vi "QTrkTest.vi"() -> ()   [LabVIEW 2015]
uses:
  QTrkLVBinding/QTrkSettings.ctl
  QTrkLVBinding/QTrkLocalizationType.ctl
  QTrkLVBinding/QTrkZCommandType.ctl
  QTrkLVBinding/QTrkDLL.vi
panel:
  in  "Number of ZLUTs":i32=1
  in  "Select dll":bool
  out "Sample img":sgl[][](graph)
  in  "stop test":bool
  out "Frame#":i32
  out "Frames/s":dbl
  in  "Testing sample count":i32=10000
  out "testing results":i32
  out "Single ZLUT plane image":sgl[][](graph)
  in  "Run":bool
  in  "stop":bool
  in  "LUT radii":cluster{"min":sgl, "max":sgl}={"min"=0.0, "max"=40.0}
  out "LUT":u8[][](graph)
  out "Generated LUT":sgl[][](graph)
  in  "Max Z":dbl=180.0
  in  "Min Z":dbl
  in  "QTrk Settings":T1={"Image width"=80, "Image height"=80, "Number of threads (CPU based)"=-1, "CUDA Device"=128, "COM Background correction factor"=2.0, "ZLUT MinRadius"=2.0, "ZLUT Radial sample density"=30.0, "ZLUT Angular sample density"=128.0, "ZLUT ROI Coverage"=32.0, "QI Iterations"=4, "QI MinRadius"=2.0, "QI Radial sample density"=32.0, "QI Angular sample density"=30.0, "QI ROI Coverage"=0.0, "QI Angular Step \nIteration Factor"=32.0, "XCOR Profile Length"=32, "XCOR Profile Width"=2, "XCOR Iterations"=5, "Gaussian 2D Fit Iterations"=8, "Gaussian 2D Sigma (pixels)"=3.0, "Downsample"=0}
  # "-2: Use all devices\n-1: Use best device"
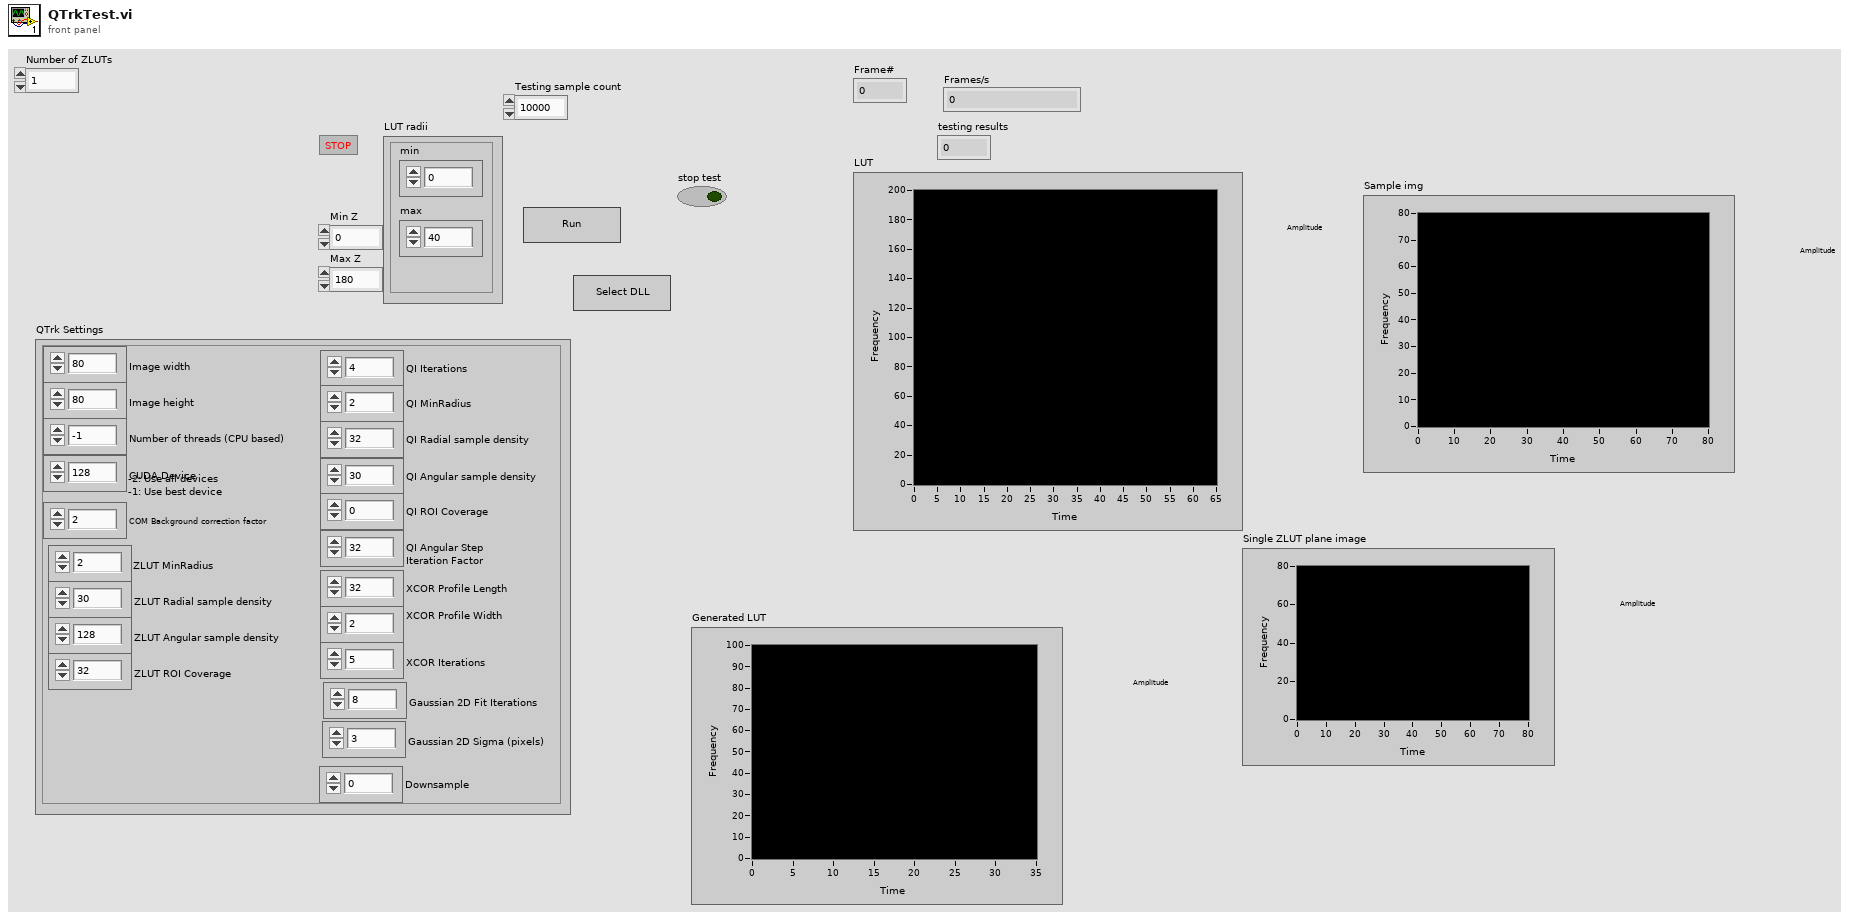
[diagram p1: front panel]
types:
  T1 = typedef "QTrkSettings.ctl" = cluster{"Image width":i32, "Image height":i32, "Number of threads (CPU based)":i32, "CUDA Device":i32, "COM Background correction factor":sgl, "ZLUT MinRadius":sgl, "ZLUT Radial sample density":sgl, "ZLUT Angular sample density":sgl, "ZLUT ROI Coverage":sgl, "QI Iterations":i32, "QI MinRadius":sgl, "QI Radial sample density":sgl, "QI Angular sample density":sgl, "QI ROI Coverage":sgl, "QI Angular Step \nIteration Factor":sgl, "XCOR Profile Length":i32, "XCOR Profile Width":i32, "XCOR Iterations":i32, "Gaussian 2D Fit Iterations":i32, "Gaussian 2D Sigma (pixels)":sgl, "Downsample":i32}
  T2 = typedef "Image Type" = u32
  T3 = typedef "IMAQ Image.ctl" = refnum<image>
  T4 = typedef "QTrkZCommandType.ctl" = enum16{"Nothing", "ComputeZ"}
  T5 = typedef "QTrkLocalizationType.ctl" = enum16{"Center-of-Mass", "1D Cross-Correlation", "Quadrant Interpolation", "Gaussian 2D MLE", "QI + ZLUTAlign", "ZLUTAlign", "QI + FourierLUT"}
  T6 = typedef "QTrkInstance.ctl" = cluster{"QTrk Pointer":u64}
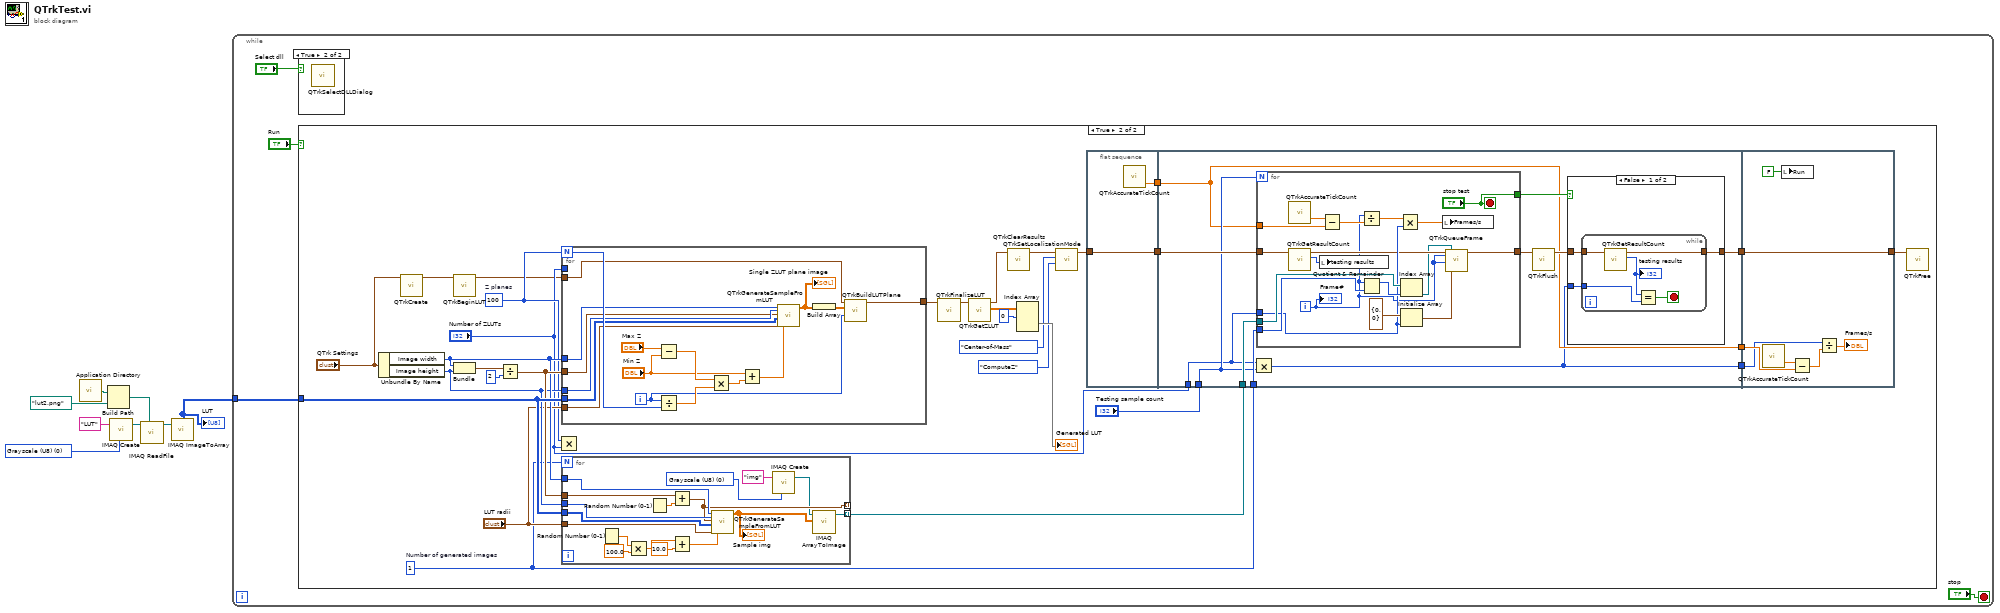
[diagram p0: block diagram]
diagram:
  w8 = T2 0 items=["Grayscale (U8)", "Grayscale (I16)", "Grayscale (SGL)", "Complex (CSG)", "RGB (U32)", "HSL (U32)", "RGB (U64)", "Grayscale (U16)"] ("Image Type")
  n1 = call <vilib>:"Application Directory.vi"() -> ("Application Directory"=w4:path)
  n2 = Build Path(base path=w4, name or relative path=path "lut2.png" ("File Path")) -> (appended path=w2:path)
  n3 = call "IMAQ Create"("Image Name"="LUT" ("String"), "Image Type"=w8) -> ("New Image"=w6:T3)  [unwired: 3 in, 1 out]
  n4 = call "IMAQ ReadFile"("File Path"=w2, "Image"=w6) -> ("Image Out"=w5:T3)  [unwired: 5 in, 4 out]
  n5 = call "IMAQ ImageToArray"("Image"=w5) -> ("Image Pixels (U8)"=w1:u8[][])  [unwired: 3 in, 4 out]
  "LUT" <- w1
  n6 = while {
    tunnel: w1 -> [w12]
    stop <- "stop" stop-if-true
    n7 = case shown="True" "Select dll" {
      frame False {
      }
      frame True {
        n8 = call "QTrkSelectDLLDialog.vi"() -> ()  [unwired: 11 in, 1 out]
      }
    }
    n9 = case shown="True" "Run" {
      tunnel: w12 -> [_ w40]
      frame False {
      }
      frame True {
        w24 = 100  # Z planes
        w29 = 1  # Number of generated images
        n10 = Unbundle By Name("QTrk Settings") -> ("Image width"=w32:i32, "Image height"=w31:i32)
        n11 = call "QTrkCreate.vi"("QTrk Settings"="QTrk Settings") -> ("QTrk Instance"=w16:T6)  [unwired: 4 in, 2 out]
        n12 = call "QTrkBeginLUT.vi"("QTrk Instance"=w16) -> ("QTrk Instance"=w15:T6)  [unwired: 5 in, 1 out]
        n13 = Bundle("Image width"=w32, "Image height"=w31) -> (w38:cluster{"Image width":i32, "Image height":i32})  [unwired: 1 in]
        n14 = Divide(x=w38, y=2 ("Image height")) -> (x/y=w36:cluster{"Image width":dbl, "Image height":dbl})
        n15 = Multiply(x=w24, y="Number of ZLUTs") -> ()  [unwired: 1 out]
        n16 = for {
          N: w24 -> [w106]
          tunnel: w36 -> [w101]
          tunnel: w15 -> [w95]
          tunnel: w32 -> [w103]
          tunnel: w31 -> [w102]
          tunnel: w40 -> [w100]
          tunnel: "LUT radii" -> [w99]
          tunnel: "Number of ZLUTs" -> [_]
          tunnel: [w91] -> w14
          i -> [w92]
          n17 = Subtract(x="Max Z", y="Min Z") -> (x-y=w105:dbl)
          n18 = Divide(x=w92, y=w106) -> (x/y=w104:dbl)
          n19 = Multiply(x=w105, y=w104) -> (x*y=w97:dbl)
          n20 = Add(x="Min Z", y=w97) -> (x+y=w96:dbl)
          n21 = call "QTrkGenerateSampleFromLUT.vi"("Width"=w103, "Height"=w102, "position"=w101, "LUT"=w100, "LUT radii"=w99, "z"=w96) -> ("image"=w94:sgl[][])  [unwired: 13 in]
          "Single ZLUT plane image" <- w94
          n22 = Build Array(w94) -> (w93:sgl[][][])
          n23 = call "QTrkBuildLUTPlane.vi"("QTrk Instance"=w95, "Bead images"=w93, "plane"=w92) -> ("QTrk Instance"=w91:T6)  [unwired: 11 in, 1 out]
        }
        n24 = for {
          N: w29 -> [_]
          tunnel: w36 -> [w124]
          tunnel: [w119] -> _ mode=indexing
          tunnel: w32 -> [w121]
          tunnel: w31 -> [w120]
          tunnel: w40 -> [w118]
          tunnel: "LUT radii" -> [w117]
          tunnel: [w110] -> w25 mode=indexing
          w112 = T2 0 items=["Grayscale (U8)", "Grayscale (I16)", "Grayscale (SGL)", "Complex (CSG)", "RGB (U32)", "HSL (U32)", "RGB (U64)", "Grayscale (U16)"] ("Image Type")
          n25 = Random Number (0-1)() -> (number: 0 to 1=w115:dbl)
          n26 = Multiply(x=w115, y=100.0) -> (x*y=w113:dbl)
          n27 = Random Number (0-1)() -> (number: 0 to 1=w123:dbl)
          n28 = Add(x=w124, y=w123) -> (x+y=w119:cluster{"Image width":dbl, "Image height":dbl})
          n29 = Add(x=w113, y=10.0) -> (x+y=w116:dbl)
          n30 = call "QTrkGenerateSampleFromLUT.vi"("Width"=w121, "Height"=w120, "position"=w119, "LUT"=w118, "LUT radii"=w117, "z"=w116) -> ("image"=w109:sgl[][])  [unwired: 13 in]
          "Sample img" <- w109
          n31 = call "IMAQ Create"("Image Name"="img", "Image Type"=w112) -> ("New Image"=w111:T3)  [unwired: 3 in, 1 out]
          n32 = call "IMAQ ArrayToImage"("Image Pixels (U8)"=w109, "Image"=w111) -> ("Image Out"=w110:T3)  [unwired: 8 in, 1 out]
        }
        n33 = call "QTrkFinalizeLUT.vi"("QTrk Instance"=w14) -> ("QTrk Instance"=w13:T6)  [unwired: 5 in, 1 out]
        n34 = call "QTrkGetZLUT.vi"("QTrk Instance (in)"=w13) -> ("zlut"=w35:sgl[][][], "QTrk Instance"=w26:T6)  [unwired: 8 in, 1 out]
        n35 = call "QTrkClearResults.vi"("QTrk Instance (in)"=w26) -> ("QTrk Instance (out)"=w20:T6)  [unwired: 9 in, 1 out]
        n36 = Index Array(array=w35, index (dim 0)=0 ("index (page)")) -> (element=→"Generated LUT":sgl[][])  [unwired: 2 in]
        n37 = call "QTrkSetLocalizationMode.vi"("Z Command"=QTrkZCommandType."ComputeZ", "2D Localization Type"=QTrkLocalizationType."Center-of-Mass", "QTrk Instance"=w20) -> ("QTrk Instance"=w19:T6)  [unwired: 8 in]
        n38 = flat-sequence {
          tunnel: w19 -> [w45]
          tunnel: [w45] -> w43
          tunnel: [w44] -> w42
          tunnel: w29 -> [w56]
          tunnel: "Testing sample count" -> [w49]
          tunnel: w43 -> [w54]
          tunnel: [w55] -> w41
          tunnel: w42 -> [w47]
          tunnel: w25 -> [w50]
          tunnel: "Number of ZLUTs" -> [w48]
          tunnel: [w47] -> w22
          tunnel: [w46] -> w21
          tunnel: [w90] -> w27
          tunnel: w41 -> [w90]
          tunnel: w22 -> [w88]
          tunnel: w21 -> [w87]
          frame #0 {
            n39 = call "QTrkAccurateTickCount.vi"() -> ("seconds"=w44:dbl)  [unwired: 2 in, 1 out]
          }
          frame #1 {
            n40 = Multiply(x=w48, y=w49) -> (x*y=w46:i32)
            n41 = for {
              N: w49 -> [_]
              tunnel: w54 -> [w81]
              tunnel: w56 -> [w83]
              tunnel: [w69] -> w52
              tunnel: ["stop test"] -> w53
              tunnel: w47 -> [w77]
              tunnel: w50 -> [w76]
              tunnel: w48 -> [w73]
              i -> [w67]
              stop <- "stop test" stop-if-true
              n42 = call "QTrkAccurateTickCount.vi"() -> ("seconds"=w71:dbl)  [unwired: 2 in, 1 out]
              n43 = call "QTrkGetResultCount.vi"("QTrk Instance"=w81) -> ("result count"=w80:i32, "QTrk Instance"=w70:T6)  [unwired: 4 in, 1 out]
              n44 = local write "testing results"(w80) -> ()
              n45 = Subtract(x=w71, y=w77) -> (x-y=w78:dbl)
              n46 = Divide(x=w67, y=w78) -> (x/y=w74:dbl)
              n47 = Quotient & Remainder(x=w67, y=w83) -> (x-y*floor(x/y)=w82:i32)  [unwired: 1 out]
              n48 = Multiply(x=w74, y=w73) -> (x*y=w72:dbl)
              n49 = Index Array(array=w76, index=w82) -> (element=w66:T3)
              n50 = Initialize Array(cluster{"X":i32, "Y":i32} {"X"=0, "Y"=0} ("ROI Position"), w73) -> (w68:cluster{"X":i32, "Y":i32}[])
              n51 = local write "Frames/s"(w72) -> ()
              n52 = call "QTrkQueueFrame.vi"("QTrk Instance"=w70, "frame#"=w67, "timestamp"=w67, "Image"=w66, "ROI Positions (corner-based)"=w68) -> ("QTrk Instance (out)"=w69:T6)  [unwired: 12 in, 2 out]
              "Frame#" <- w67
            }
            n53 = call "QTrkFlush.vi"("QTrk Instance"=w52) -> ("QTrk Instance (out)"=w51:T6)  [unwired: 9 in, 1 out]
            n54 = case shown="False" w53 {
              tunnel: w51 -> [w59 w65]
              tunnel: [w58 w65] -> w55
              tunnel: w46 -> [w57 _]
              frame False {
                n55 = while {
                  tunnel: w59 -> [w60]
                  tunnel: [w64] -> w58
                  tunnel: w57 -> [w62]
                  stop <- w61 stop-if-true
                  n56 = call "QTrkGetResultCount.vi"("QTrk Instance"=w60) -> ("result count"=w63:i32, "QTrk Instance"=w64:T6)  [unwired: 4 in, 1 out]
                  "testing results" <- w63
                  n57 = Equal?(x=w63, y=w62) -> (x = y?=w61:bool)
                }
              }
              frame True {
              }
            }
          }
          frame #2 {
            n58 = call "QTrkAccurateTickCount.vi"() -> ("seconds"=w84:dbl)  [unwired: 2 in, 1 out]
            n59 = local write "Run"(FALSE ("Run")) -> ()
            n60 = Subtract(x=w84, y=w88) -> (x-y=w86:dbl)
            n61 = Divide(x=w87, y=w86) -> (x/y=→"Frames/s":dbl)
          }
        }
        n62 = call "QTrkFree.vi"("QTrk Instance"=w27) -> ()  [unwired: 6 in, 1 out]
      }
    }
  }
